vi "crc16-ccitt from string.vi"(8 "error in (no error)":errorcluster, 11 "String":string) -> (0 "error out":errorcluster, 3 "CRC Out":i32 format="0x%x")   [LabVIEW 2016]
uses:
  Inline CRC/CRC SubVIs/Wrappers/CRC-16-CCITT-0xFFFF.vi
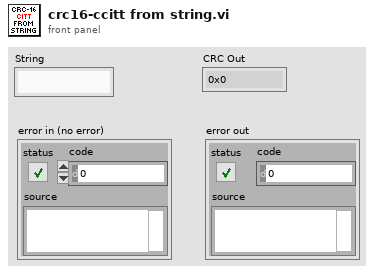
[diagram p1: front panel]
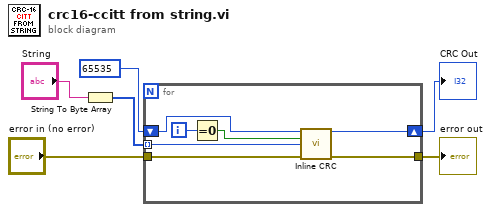
[diagram p0: block diagram]
diagram:
  n1 = String To Byte Array(string="String") -> (unsigned byte array=w2:u8[])
  n2 = for {
    tunnel: "error in (no error)" -> [w13]
    shift-right: [w11] -> w6
    shift-left: 65535 -> [w12]
    tunnel: [w10] -> w5
    tunnel: w2 -> [w9] mode=indexing
    i -> [w8]
    n3 = Equal To 0?(x=w8) -> (x = 0?=w7:bool)
    n4 = call-poly "Inline CRC.vi"("CRC In"=w12, "Reset"=w7, "Data"=w9, "error in (no error)"=w13) -> ("CRC"=w11:u16, "error out"=w10:errorcluster)  [unwired: 10 in]
  }
  "CRC Out" <- w6
  "error out" <- w5
